vi "Weather JSON to cluster.vi"(11 "JSON status":string) -> (3 "Weather160":T1)   [LabVIEW 2012]
panel:
  # "O nome e o tipo de dados dos\ncontroles do indicador \"JSON cluster\" devem ser iguais aos \nkeywords e valores da string \"JSON status\"."
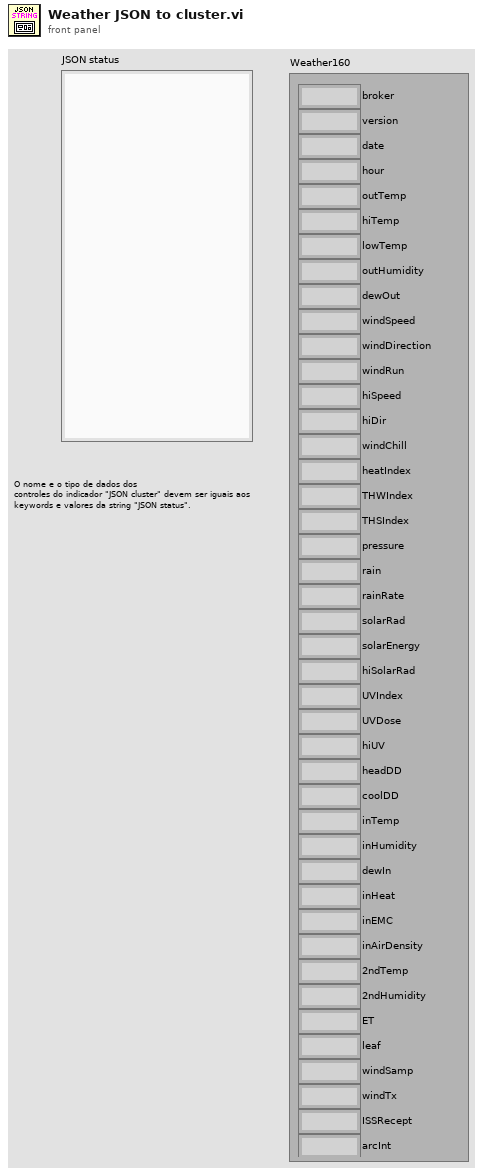
[diagram p1: front panel]
types:
  T1 = cluster{"broker":string, "version":string, "date":string, "hour":string, "outTemp":string, "hiTemp":string, "lowTemp":string, "outHumidity":string, "dewOut":string, "windSpeed":string, "windDirection":string, "windRun":string, "hiSpeed":string, "hiDir":string, "windChill":string, "heatIndex":string, "THWIndex":string, "THSIndex":string, "pressure":string, "rain":string, "rainRate":string, "solarRad":string, "solarEnergy":string, "hiSolarRad":string, "UVIndex":string, "UVDose":string, "hiUV":string, "headDD":string, "coolDD":string, "inTemp":string, "inHumidity":string, "inHeat":string, "inEMC":string, "inAirDensity":string, "2ndTemp":string, "2ndHumidity":string, "ET":string, "leaf":string, "windSamp":string, "windTx":string, "ISSRecept":string, "dewIn":string, "arcInt":string}
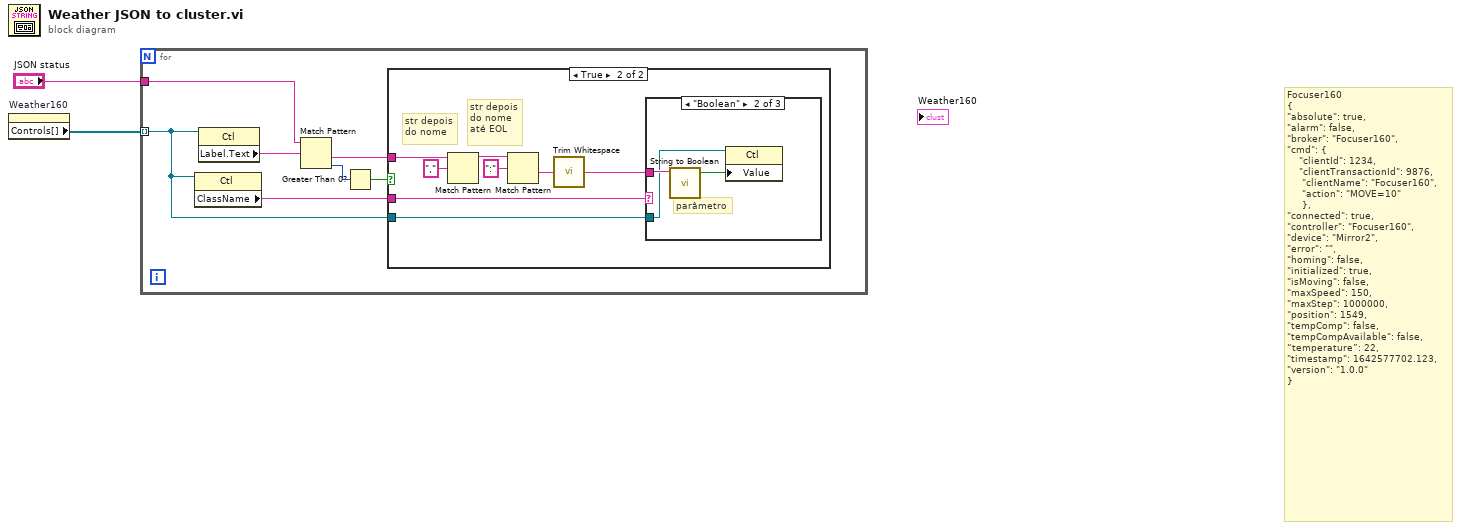
[diagram p0: block diagram]
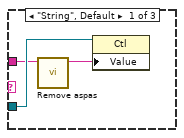
[diagram p3: hidden frame]
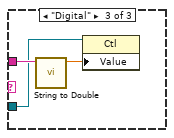
[diagram p4: hidden frame]
diagram:
  # "Focuser160\n{\n\"absolute\": true,\n\"alarm\": false,\n\"broker\": \"Focuser160\",\n\"cmd\": {\n    \"clientId\": 1234,\n    \"clientTransactionId\": 9876,\n     \"clientName\": \"Focuser160\",\n     \"action\": \"MOVE=10\"\n     },\n\"connected\": true,\n\"controller\": \"Focuser160\",\n\"device\": \"Mirror2\",\n\"error\": \"\",\n\"homing\": false,\n\"initialized\": true,\n\"isMoving\": false,\n\"maxSpeed\": 150,\n\"maxStep\": 1000000,\n\"position\": 1549,\n\"tempComp\": false,\n\"tempCompAvailable\": false,\n“temperature”: 22,\n\"timestamp\": 1642577702.123,\n\"version\": \"1.0.0\"\n}"
  n1 = property on="Weather160" class="Clust (strict)"() -> ("Controls[]"=w1:refnum<vi>[])  [unwired: 2 in, 2 out]
  n2 = for {
    tunnel: w1 -> [w3] mode=indexing
    tunnel: "JSON status" -> [w6]
    n3 = property class="Ctl"(reference=w3) -> ("ClassName"=w4:string)  [unwired: 1 in, 2 out]
    n4 = property class="Ctl"(reference=w3) -> ("Label.Text"=w9:string)  [unwired: 1 in, 2 out]
    n5 = Match Pattern(string=w6, regular expression=w9) -> (after substring=w5:string, offset past match=w8:i32)  [unwired: 1 in, 2 out]
    n6 = Greater Than 0?(x=w8) -> (x > 0?=w7:bool)
    n7 = case shown="True" w7 {
      tunnel: w5 -> [_ w17]
      tunnel: w4 -> [_ w13]
      tunnel: w3 -> [_ w12]
      frame False {
      }
      frame True {
        # "str depois\ndo nome\naté EOL"
        # "str depois\ndo nome"
        n8 = Match Pattern(string=w17, regular expression=",") -> (before substring=w15:string)  [unwired: 1 in, 3 out]
        n9 = Match Pattern(string=w15, regular expression=":") -> (after substring=w10:string)  [unwired: 1 in, 3 out]
        n10 = call <vilib>:"Trim Whitespace.vi"("string"=w10) -> ("trimmed string"=w11:string)  [unwired: 1 in]
        n11 = case shown="\"Boolean\"" w13 {
          tunnel: w11 -> [w19 w23 w26]
          tunnel: w12 -> [w20 w22 w25]
          frame "String", Default {
            n12 = call "Remove aspas.vi"("textoComAspas"=w19) -> ("textoEntreAspas"=w18:string)  [unwired: 10 in]
            n13 = property class="Ctl"(reference=w20, "Value"=w18) -> ()  [unwired: 1 in, 2 out]
          }
          frame "Boolean" {
            # "parâmetro"
            n14 = call "String to Boolean.vi"("booleanString"=w23) -> ("state"=w21:bool)  [unwired: 10 in]
            n15 = property class="Ctl"(reference=w22, "Value"=w21) -> ()  [unwired: 1 in, 2 out]
          }
          frame "Digital" {
            n16 = call "String to Double.vi"("fractionalString"=w26) -> ("value"=w24:dbl)  [unwired: 10 in]
            n17 = property class="Ctl"(reference=w25, "Value"=w24) -> ()  [unwired: 1 in, 2 out]
          }
        }
      }
    }
  }
